vi "CompilerLoadPulseTexts.vi"(4 "compile settings":T1={"Python Path"=path "", "Main File"="makesequence.py", "Meta File"="makesequence.py", "Aux File"="makesequence.py", "Pre File"="metascript.txt"}) -> (0 "AuxCode 2":string, 1 "MetaCode 2":string, 2 "Maincode 2":string)   [LabVIEW 2019]
uses:
  PulseCompiler/CompilerSettings.ctl
panel:
  out "error out 3":errorcluster
  out "error out 2":errorcluster
  out "error out":errorcluster
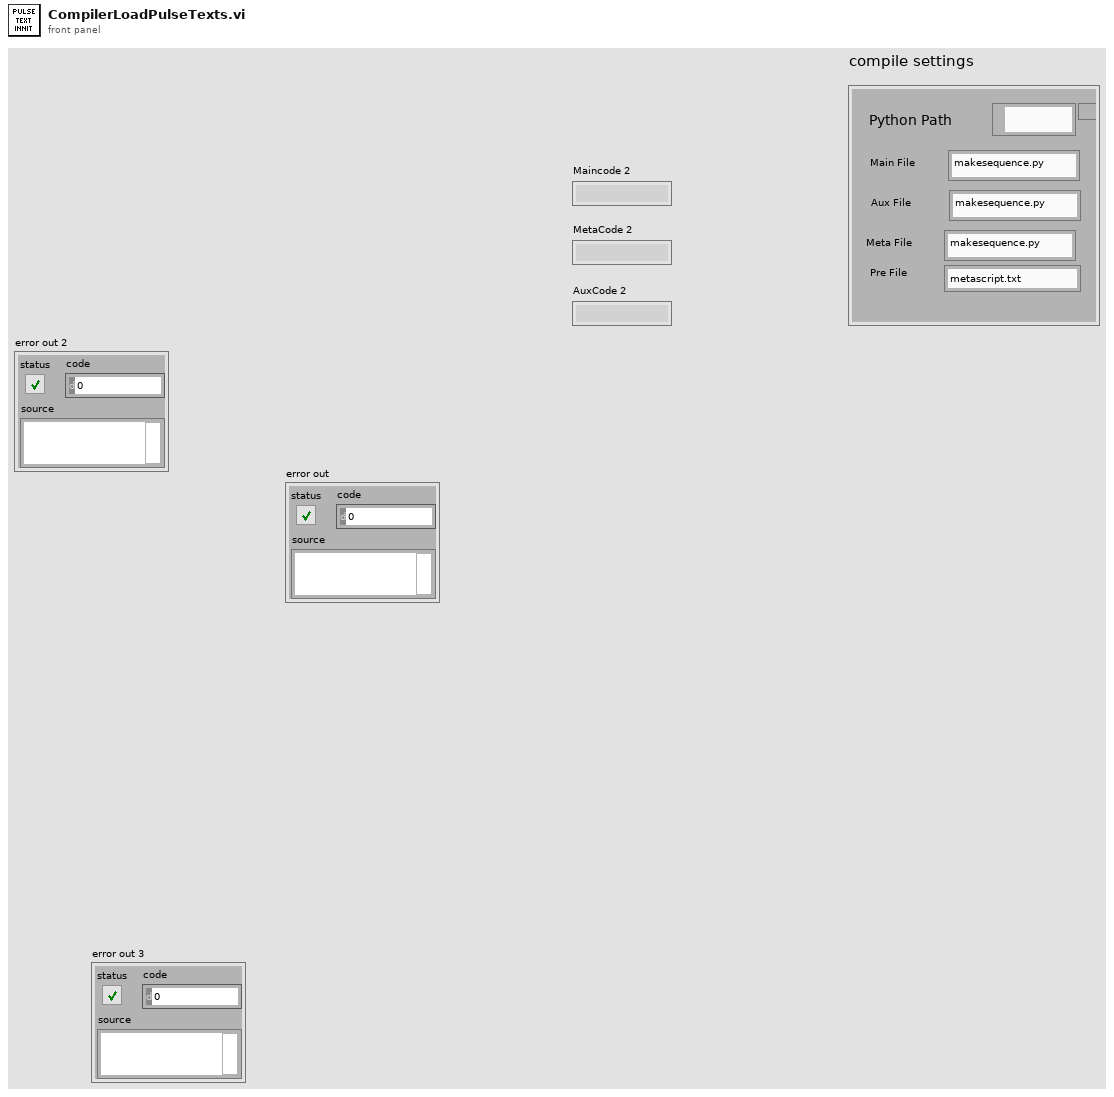
[diagram p1: front panel]
types:
  T1 = typedef "CompilerSettings.ctl" = cluster{"Python Path":path, "Main File":string, "Meta File":string, "Aux File":string, "Pre File":string}
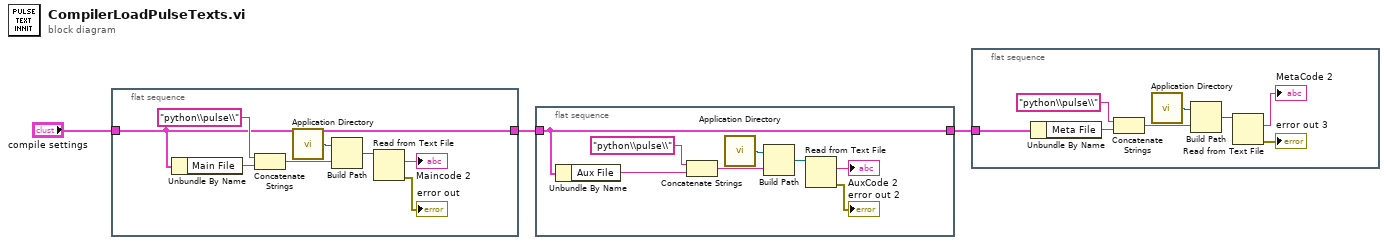
[diagram p0: block diagram]
diagram:
  n1 = flat-sequence {
    tunnel: "compile settings" -> [w5]
    tunnel: [w5] -> w2
    frame #0 {
      n2 = Unbundle By Name(w5) -> ("Main File"=w8:string)
      n3 = Concatenate Strings("python\\pulse\\" ("string"), w8) -> (w10:string)
      n4 = call <vilib>:"Application Directory.vi"() -> ("Application Directory"=w11:path)
      n5 = Build Path(base path=w11, name or relative path=w10) -> (appended path=w7:path)
      n6 = Read from Text File(file (use dialog)=w7) -> (text=→"Maincode 2":string, error out=→"error out":errorcluster)  [unwired: 3 in, 2 out]
    }
  }
  n7 = flat-sequence {
    tunnel: w2 -> [w13]
    tunnel: [w13] -> w1
    frame #0 {
      n8 = Unbundle By Name(w13) -> ("Aux File"=w16:string)
      n9 = Concatenate Strings("python\\pulse\\" ("string"), w16) -> (w18:string)
      n10 = call <vilib>:"Application Directory.vi"() -> ("Application Directory"=w19:path)
      n11 = Build Path(base path=w19, name or relative path=w18) -> (appended path=w15:path)
      n12 = Read from Text File(file (use dialog)=w15) -> (text=→"AuxCode 2":string, error out=→"error out 2":errorcluster)  [unwired: 3 in, 2 out]
    }
  }
  n13 = flat-sequence {
    tunnel: w1 -> [w21]
    frame #0 {
      n14 = Unbundle By Name(w21) -> ("Meta File"=w24:string)
      n15 = Concatenate Strings("python\\pulse\\" ("string"), w24) -> (w26:string)
      n16 = call <vilib>:"Application Directory.vi"() -> ("Application Directory"=w27:path)
      n17 = Build Path(base path=w27, name or relative path=w26) -> (appended path=w23:path)
      n18 = Read from Text File(file (use dialog)=w23) -> (text=→"MetaCode 2":string, error out=→"error out 3":errorcluster)  [unwired: 3 in, 2 out]
    }
  }
